vi "setUp.vi"(8 "error in (no error)":errorcluster, 11 "reference in":refnum<class "FPGA Addon Scalar Bitpacking Unit Tests.lvclass">) -> (0 "error out":errorcluster, 3 "reference out":refnum<class "FPGA Addon Scalar Bitpacking Unit Tests.lvclass">)   [LabVIEW 2018, in "FPGA Addon Scalar Bitpacking Unit Tests.lvclass"]
doc: "setUp runs prior to the test method during test execution. Use this method to initialize any object data required by your tests."
uses:
  FPGA Addon Scalar Bitpacking Unit Tests.lvclass
  C:/Program Files (x86)/National Instruments/LabVIEW 2018/vi.lib/addons/_JKI Toolkits/VI Tester/TestCase.llb/TestCase.lvclass
  FPGA Addon Scalar Bitpacking Unit Tests.lvclass/FPGA Addon Scalar Bitpacking Unit Tests.ctl
  <vilib>/addons/_JKI Toolkits/VI Tester/TestCase.llb/TestCase.lvclass
  FPGA Addon Test Class/FPGA Addon Test Class.lvclass
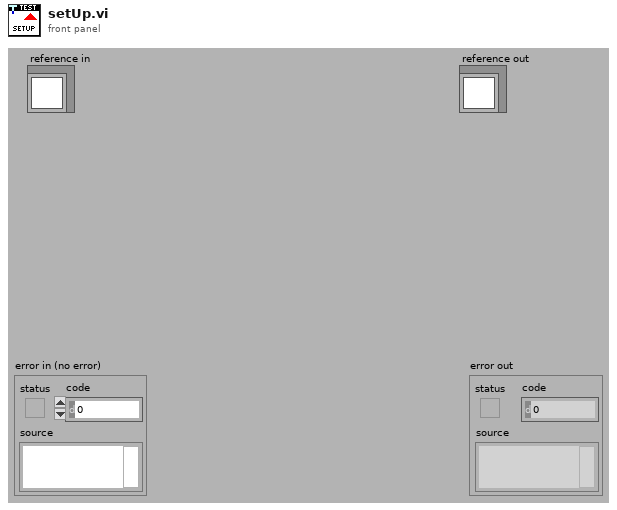
[diagram p1: front panel]
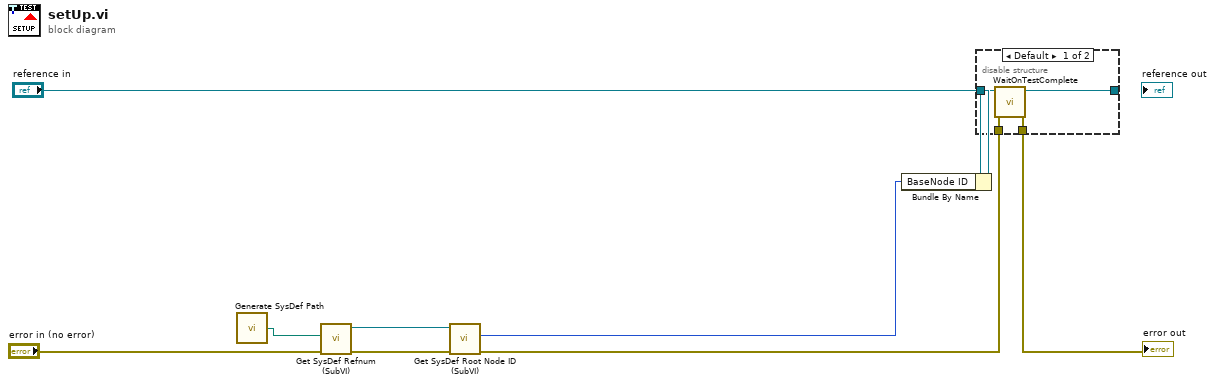
[diagram p0: block diagram]
diagram:
  n1 = call "Generate SysDef Path.vi"() -> ("System Definition path"=w1:path)
  n2 = call "Get SysDef Refnum (SubVI).vi"("error in (no error)"="error in (no error)", "System Definition path"=w1) -> ("error out"=w5:errorcluster, "SysDef Refnum out"=w3:refnum<k24>)  [unwired: 8 in]
  n3 = call "Get SysDef Root Node ID (SubVI).vi"("error in (no error)"=w5, "SysDef Refnum In"=w3) -> ("error out"=w4:errorcluster, "Root NodeID Out"=w2:u64)  [unwired: 7 in, 1 out]
  n4 = Bundle By Name(cluster="reference in", "BaseNode ID"=w2) -> (w8:refnum<class "FPGA Addon Scalar Bitpacking Unit Tests.lvclass">)
  n5 = disable-structure shown="Default" {
    disable-tunnel: w4 -> [w13 w14]
    disable-tunnel: [w12 w14] -> w9
    disable-tunnel: [w11 w15] -> _
    disable-tunnel: w8 -> [w10 w15]
    frame condition #0 (active) {
      n6 = call <vilib>:"WaitOnTestComplete.vi"("error in (no error)"=w13, "TestCase in"=w10) -> ("error out"=w12:errorcluster, "TestCase out"=w11:refnum<class "FPGA Addon Scalar Bitpacking Unit Tests.lvclass">)  [unwired: 8 in]
    }
    frame condition #1 {
    }
  }
  "error out" <- w9
